vi "Get Class Attributes.vi"(8 "error in (no error)":errorcluster, 11 "New Getter Dialog In":refnum<class "New Getter Dialog.lvclass">) -> (0 "error out":errorcluster, 3 "New Getter Dialog Out":refnum<class "New Getter Dialog.lvclass">)   [LabVIEW 2020, in "Method Generation.lvlib" / "New Getter Dialog.lvclass"]
uses:
  New Getter Dialog.lvclass
  New Getter Dialog.lvclass/New Getter Dialog.ctl
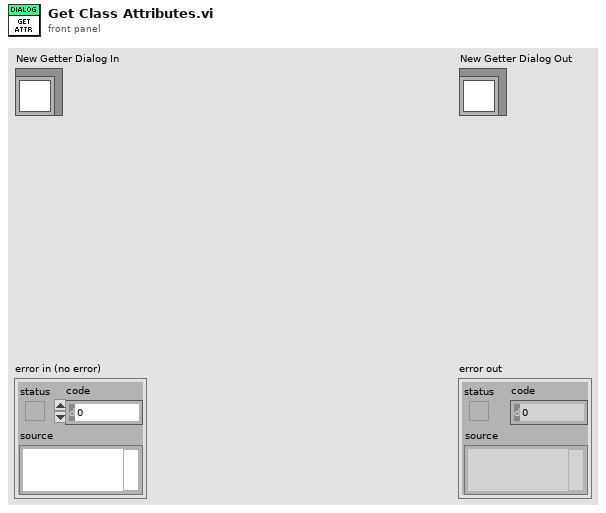
[diagram p1: front panel]
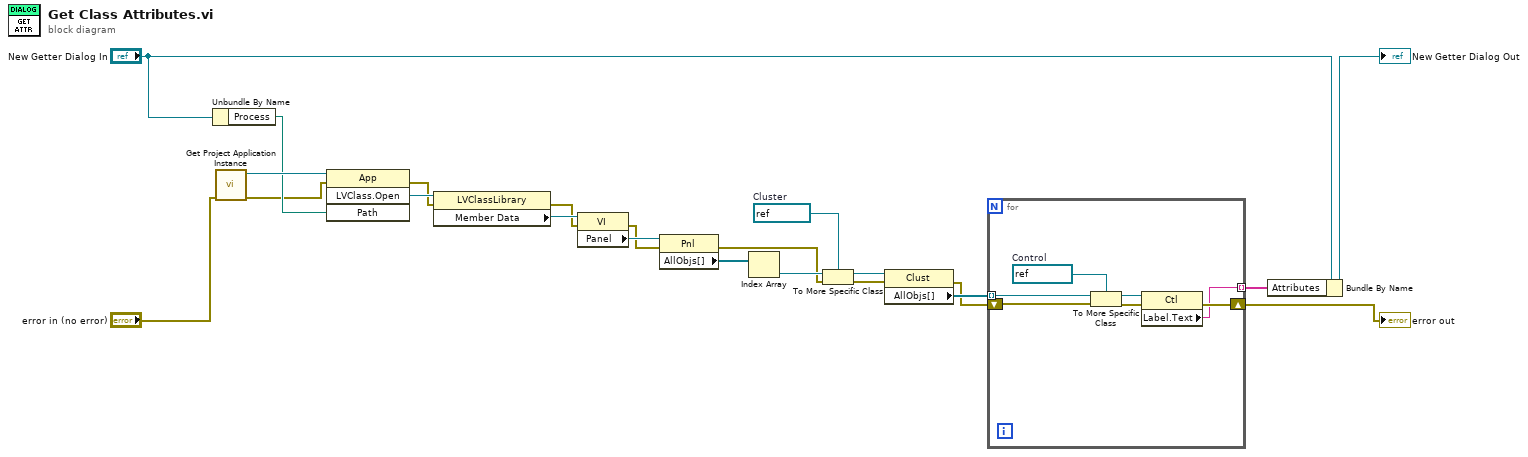
[diagram p0: block diagram]
diagram:
  w13 = refnum<vi> refnum  # Cluster
  n1 = Unbundle By Name("New Getter Dialog In") -> ("Process"=w21:path)
  n2 = call "Get Project Application Instance.vi"("error in (no error)"="error in (no error)") -> ("error out"=w20:errorcluster, "Application out"=w22:refnum<vi>)  [unwired: 9 in]
  n3 = invoke class="App" method="LVClass.Open"(reference=w22, error in=w20, "Path"=w21) -> (error out=w2:errorcluster, "LVClass.Open"=w18:refnum<vi>)  [unwired: 1 in, 2 out]
  n4 = property class="LVClassLibrary"(reference=w18, error in=w2) -> (error out=w3:errorcluster, "Member Data"=w17:refnum<vi>)  [unwired: 1 out]
  n5 = property class="VI"(reference=w17, error in=w3) -> (error out=w4:errorcluster, "Panel"=w16:refnum<vi>)  [unwired: 1 out]
  n6 = property class="Pnl"(reference=w16, error in=w4) -> (error out=w5:errorcluster, "AllObjs[]"=w15:refnum<vi>[])  [unwired: 1 out]
  n7 = Index Array(array=w15) -> (element=w14:refnum<vi>)  [unwired: 1 in]
  n8 = To More Specific Class(target class=w13, reference=w14, error in=w5) -> (specific class reference=w11:refnum<vi>, error out=w6:errorcluster)
  n9 = property class="Clust"(reference=w11, error in=w6) -> (error out=w7:errorcluster, "AllObjs[]"=w12:refnum<vi>[])  [unwired: 1 out]
  n10 = for {
    tunnel: w12 -> [w29] mode=indexing
    shift-right: [w26] -> w8
    shift-left: w7 -> [w24]
    tunnel: [w23] -> w1 mode=indexing
    w27 = refnum<vi> refnum  # Control
    n11 = To More Specific Class(target class=w27, reference=w29, error in=w24) -> (specific class reference=w28:refnum<vi>, error out=w25:errorcluster)
    n12 = property class="Ctl"(reference=w28, error in=w25) -> (error out=w26:errorcluster, "Label.Text"=w23:string)  [unwired: 1 out]
  }
  "error out" <- w8
  n13 = Bundle By Name(cluster="New Getter Dialog In", "Attributes"=w1) -> (→"New Getter Dialog Out":refnum<class "New Getter Dialog.lvclass">)
